vi "Build FEFF Filter Query.vi"(8 "error in (no error)":errorcluster, 11 "Post Analysis in":refnum<class "Post Analysis.lvclass">) -> (0 "error out":errorcluster, 2 "Query":string, 3 "Post Analysis out":refnum<class "Post Analysis.lvclass">)   [LabVIEW 2023, in "Data Analysis.lvlib" / "Post Analysis.lvlib" / "Post Analysis.lvclass"]
uses:
  Post Analysis.lvclass
  Post Analysis.lvclass/Post Analysis.ctl
panel:
  in  "Stop Test Cycle":string(combo) caption="Test Cycle"
  in  "Start Test Cycle":string(combo) caption="Test Cycle"
  in  "Test Mode":string(combo)
  in  "Test Socket":string(combo)
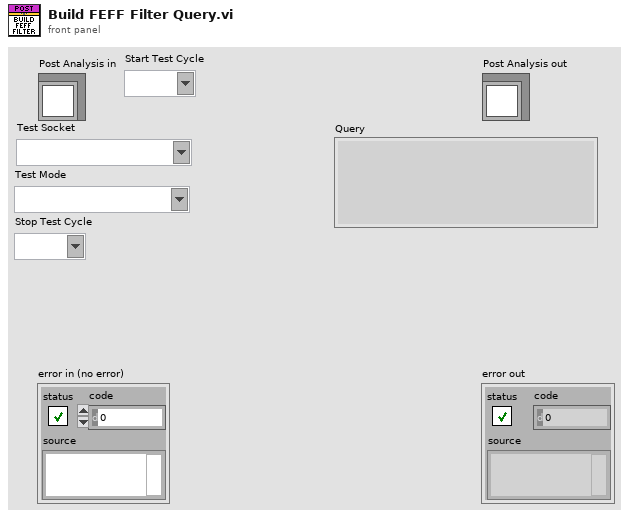
[diagram p1: front panel]
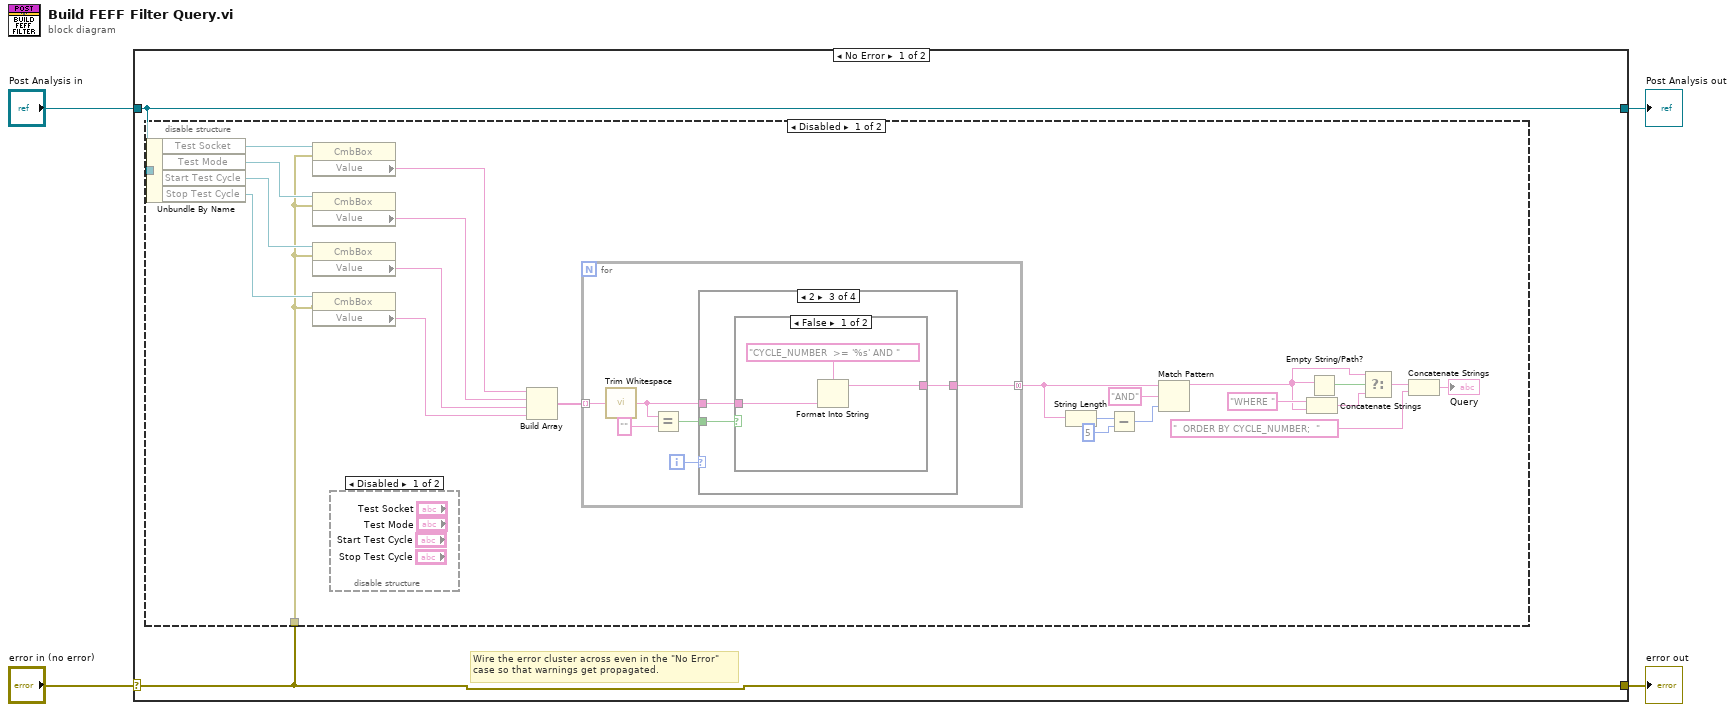
[diagram p0: block diagram]
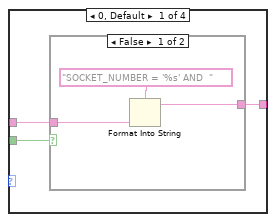
[diagram p3: hidden frame]
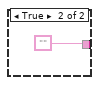
[diagram p4: hidden frame]
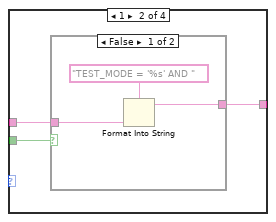
[diagram p5: hidden frame]
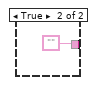
[diagram p6: hidden frame]
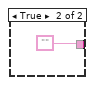
[diagram p7: hidden frame]
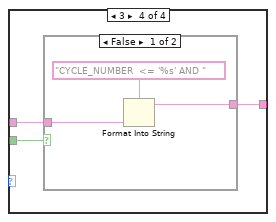
[diagram p8: hidden frame]
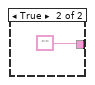
[diagram p9: hidden frame]
diagram:
  n1 = case shown="No Error" "error in (no error)" {
    selector: "error in (no error)" -> [w5 w65]
    tunnel: [w5 w65] -> w3
    tunnel: [w6 w64] -> w1
    tunnel: "Post Analysis in" -> [w6 w64]
    frame No Error {
      # "Wire the error cluster across even in the \"No Error\"\ncase so that warnings get propagated."
      n2 = disable-structure shown="Disabled" {
        disable-tunnel: w6 -> [w16 _]
        disable-tunnel: w5 -> [w11 _]
        frame Disabled {
          n3 = Unbundle By Name(w16) -> ("Test Socket"=w15:refnum<vi>, "Test Mode"=w14:refnum<vi>, "Start Test Cycle"=w13:refnum<vi>, "Stop Test Cycle"=w12:refnum<vi>)
          n4 = property class="CmbBox"(reference=w15, error in=w11) -> ("Value"=w7:string)  [unwired: 2 out]
          n5 = property class="CmbBox"(reference=w14, error in=w11) -> ("Value"=w8:string)  [unwired: 2 out]
          n6 = property class="CmbBox"(reference=w13, error in=w11) -> ("Value"=w9:string)  [unwired: 2 out]
          n7 = property class="CmbBox"(reference=w12, error in=w11) -> ("Value"=w10:string)  [unwired: 2 out]
          n8 = disable-structure shown="Disabled" {
            frame Disabled {
            }
            frame Enabled {
            }
          }
          n9 = Build Array(w7, w8, w9, w10) -> (w29:string[])
          n10 = for {
            tunnel: w29 -> [w35] mode=indexing
            tunnel: [w30] -> w20 mode=concatenating
            i -> [w33]
            n11 = call <vilib>:"Trim Whitespace.vi"("string"=w35) -> ("trimmed string"=w32:string)  [unwired: 1 in]
            n12 = Equal?(x=w32, y="") -> (x = y?=w31:bool)
            n13 = case shown="2" w33 {
              tunnel: w32 -> [w37 w44 w51 w58]
              tunnel: w31 -> [w38 w45 w52 w59]
              tunnel: [w36 w43 w50 w57] -> w30
              frame 0, Default {
                n14 = case shown="False" w38 {
                  tunnel: w37 -> [w40 _]
                  tunnel: [w39 ""] -> w36
                  frame False {
                    n15 = Format Into String(format string="SOCKET_NUMBER = '%s' AND  ", w40) -> (resulting string=w39:string)  [unwired: 2 in, 1 out]
                  }
                  frame True {
                  }
                }
              }
              frame 1 {
                n16 = case shown="False" w45 {
                  tunnel: w44 -> [w47 _]
                  tunnel: [w46 ""] -> w43
                  frame False {
                    n17 = Format Into String(format string="TEST_MODE = '%s' AND ", w47) -> (resulting string=w46:string)  [unwired: 2 in, 1 out]
                  }
                  frame True {
                  }
                }
              }
              frame 2 {
                n18 = case shown="False" w52 {
                  tunnel: w51 -> [w54 _]
                  tunnel: [w53 ""] -> w50
                  frame False {
                    n19 = Format Into String(format string="CYCLE_NUMBER  >= '%s' AND ", w54) -> (resulting string=w53:string)  [unwired: 2 in, 1 out]
                  }
                  frame True {
                  }
                }
              }
              frame 3 {
                n20 = case shown="False" w59 {
                  tunnel: w58 -> [w61 _]
                  tunnel: [w60 ""] -> w57
                  frame False {
                    n21 = Format Into String(format string="CYCLE_NUMBER  <= '%s' AND ", w61) -> (resulting string=w60:string)  [unwired: 2 in, 1 out]
                  }
                  frame True {
                  }
                }
              }
            }
          }
          n22 = String Length(string=w20) -> (length=w19:i32)
          n23 = Subtract(x=w19, y=5) -> (x-y=w17:i32)
          n24 = Match Pattern(string=w20, regular expression="AND", offset (0)=w17) -> (before substring=w21:string)  [unwired: 3 out]
          n25 = Concatenate Strings("WHERE ", w21) -> (w26:string)
          n26 = Empty String/Path?(string/path=w21) -> (empty?=w28:bool)
          n27 = Select(t=w21, s=w28, f=w26) -> (s? t:f=w25:string)
          n28 = Concatenate Strings(w25, "  ORDER BY CYCLE_NUMBER;  ") -> (→"Query":string)
        }
        frame Enabled {
        }
      }
    }
    frame Error {
    }
  }
  "error out" <- w3
  "Post Analysis out" <- w1
